vi "MainPageView.vi"() -> ()   [LabVIEW 2019]
uses:
  5219f83a-bb3a-43cd-b5ef-a6428703de02.vi
  bfe8fdff-ee4d-4ca5-9305-d53f92f2cf8d.vi
  e43f5a57-97c3-4510-b462-1dcb9a512c17.vi
  53e623ed-4a67-4f72-830e-33223b212eec.vi
  eefd14c2-1e60-472f-994b-7173b29c75b6.vi
  318ac530-f13b-4ebc-a1dc-b4da8ab9507f.vi
  911cadfa-6fc0-46bf-988e-f112db61373a.vi
  c961a98e-d49d-4477-bf1b-ce74dc2a816e.vi
  <vilib>/numeric/Random Number (Range) U64.vi
  <vilib>/numeric/sub_Random U32.vi
panel:
  in  "反馈延迟":u32=5 caption="侦听反馈延迟" max=5000 format="%.0f ms"
  in  "启用反馈？":bool
  in  "主发等待":u32=5 caption="发送后等待反馈" min=5 max=10000 format="%.0f ms"
  in  "等待延迟":u32=5 caption="侦听等待频率" min=5 max=5000 format="%.0f ms"
  out "循环引用":refnum<vi>
  out "计算后字符串":string
  out "预览":string
  in  "末尾":bool=TRUE
  in  "发送":bool
  in  "发送输入":string
  in  "寄存器重置":T1={"重置模式"=enum."址值一致", "数量"=1500, "值"=0}
  in  "清除记录":bool
  in  "清除显示":bool
  in  "寄存器重置":bool
  in  "选项卡":enum32{"被询问接收显示", "主动命令发收显示", "备注/解释/其它"}(tab)
  out "16":string[][](table) caption="功能码 16（0X10）"
  out "06":string[][](table) caption="功能码 06"
  out "03":string[][](table) caption="功能码 03"
  out "错误报文":string[][](table) caption="MB RTU 解析失败/其它 报文"
  in  "03去重":bool=TRUE caption="03指令去重？"
  out "主动接收":string[][](table) caption="接收"
  out "主动发送":string[][](table) caption="发送"
  out "连接通讯状态":bool
  out "报文流水显示":string
  in  "记录上限设置":u16=200 format="%d 条"
  out "模拟寄存器":u16[](array[numeric])
  out "连接提示":string
  out "连接模式":string
  out "显示连接":string
  in  "停止":bool
  # "发送时末尾添加?"
  # "+0"
  # "+5"
  # "+10"
  # "+15"
  # "ModbusRTU\n内置解析范围，当前针对功能码：03 06 16(十进制数)\n接收只针对询问报文的拆解，其它类型会被划分为未知命令\n\n示例格式(00代表U8字符，0000即U16字符，十六进制字符串显示)\n03询问：    01          03        0000         0001        XXXX \n            通讯地址  功能码  寄存器地址  需求数据量  CRC16\n03反馈：    01          03          00           0000 ... 0000         XXXX \n            通讯地址  功能码  数据字节量  数据段(根据询问反馈)  CRC16\n    **字节量代表U8数量，是数据量（U16字）的两倍。\n06下发/反馈  一致\n                01         06          0000      0000    XXXX\n            通讯地址  功能码  寄存器地址  写入值  CRC16\n16下发\n               01           10        0000        0001        02        0000     XXXX\n            通讯地址  功能码  寄存器地址  数据量  数据字节量  数据段  CRC16 \n16反馈\n               01          10        0000       0001    XXXX\n           通讯地址  功能码  寄存器地址  数据量  CRC16\n\n接收报文解析，只针对于询问/下发做拆解反馈"
  # "关于几个时间设置说明\n  通讯侦听部分是由\n    被动侦听-被动反馈-*主动发送命令-*主动命令反馈\n*指只有当前选中的连接执行，且无命令会忽略\n侦听等待频率-被动侦听等待超时设置\n发送后等待反馈-发送命令后等待反馈超时设置\n\n串口自发自收情况下，发送后无法获取反馈，需要测试修改\n正在测试中"
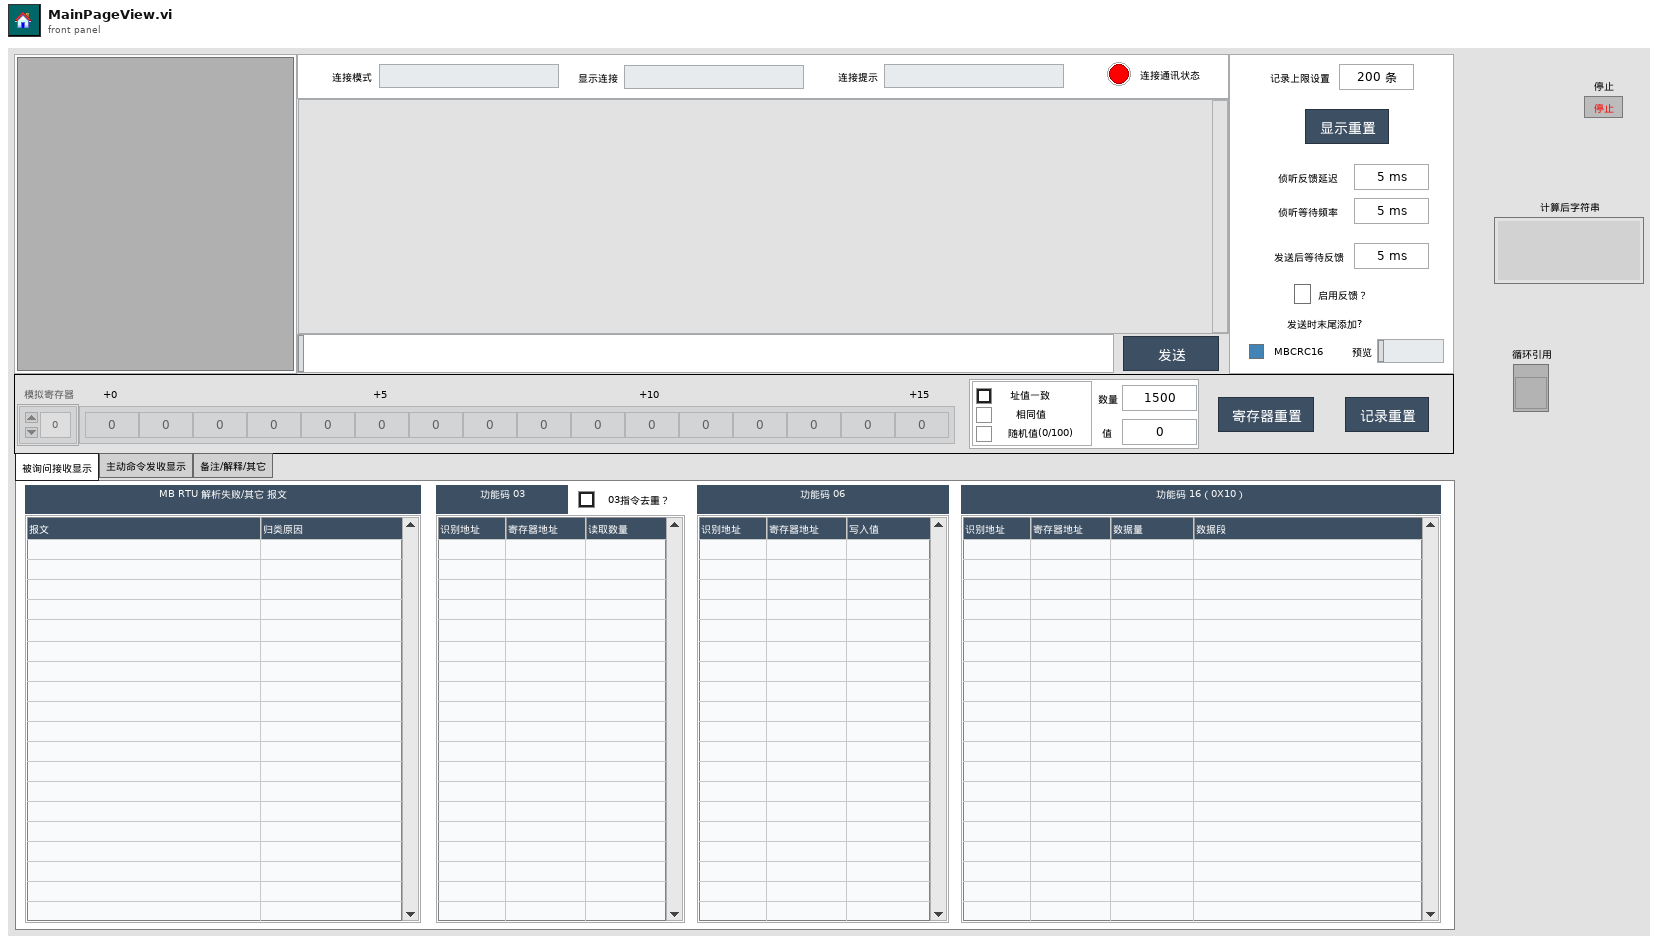
[diagram p1: front panel]
types:
  T1 = cluster{"重置模式":enum32{"址值一致", "相同值", "随机值(0/100)"}, "数量":u16, "值":u16}
  T2 = typedef "队列枚举.ctl" = enum16{"ini", "读", "写"}
  T3 = cluster{"识别名称":string, "记录":cluster{"通讯状态":bool, "记录上限":dbl, "报文记录":string[]}}
  T4 = enum16{"ini", "增", "删", "查", "改-通讯状态", "改-记录上限", "增-报文", "清空报文记录", "清空全部记录"}
  T5 = enum8{"Enabled", "Disabled", "Disabled and Grayed Out"}
  T6 = cluster{"无记录?":bool, "记录":cluster{"通讯状态":bool, "记录上限":dbl, "报文记录":string[][], "03类（被收）":string[], "06类（被收）":string[], "16类（被收）":string[], "主动发送记录":string[][], "主动接收记录":string[][], "无法识别记录":string[][]}}
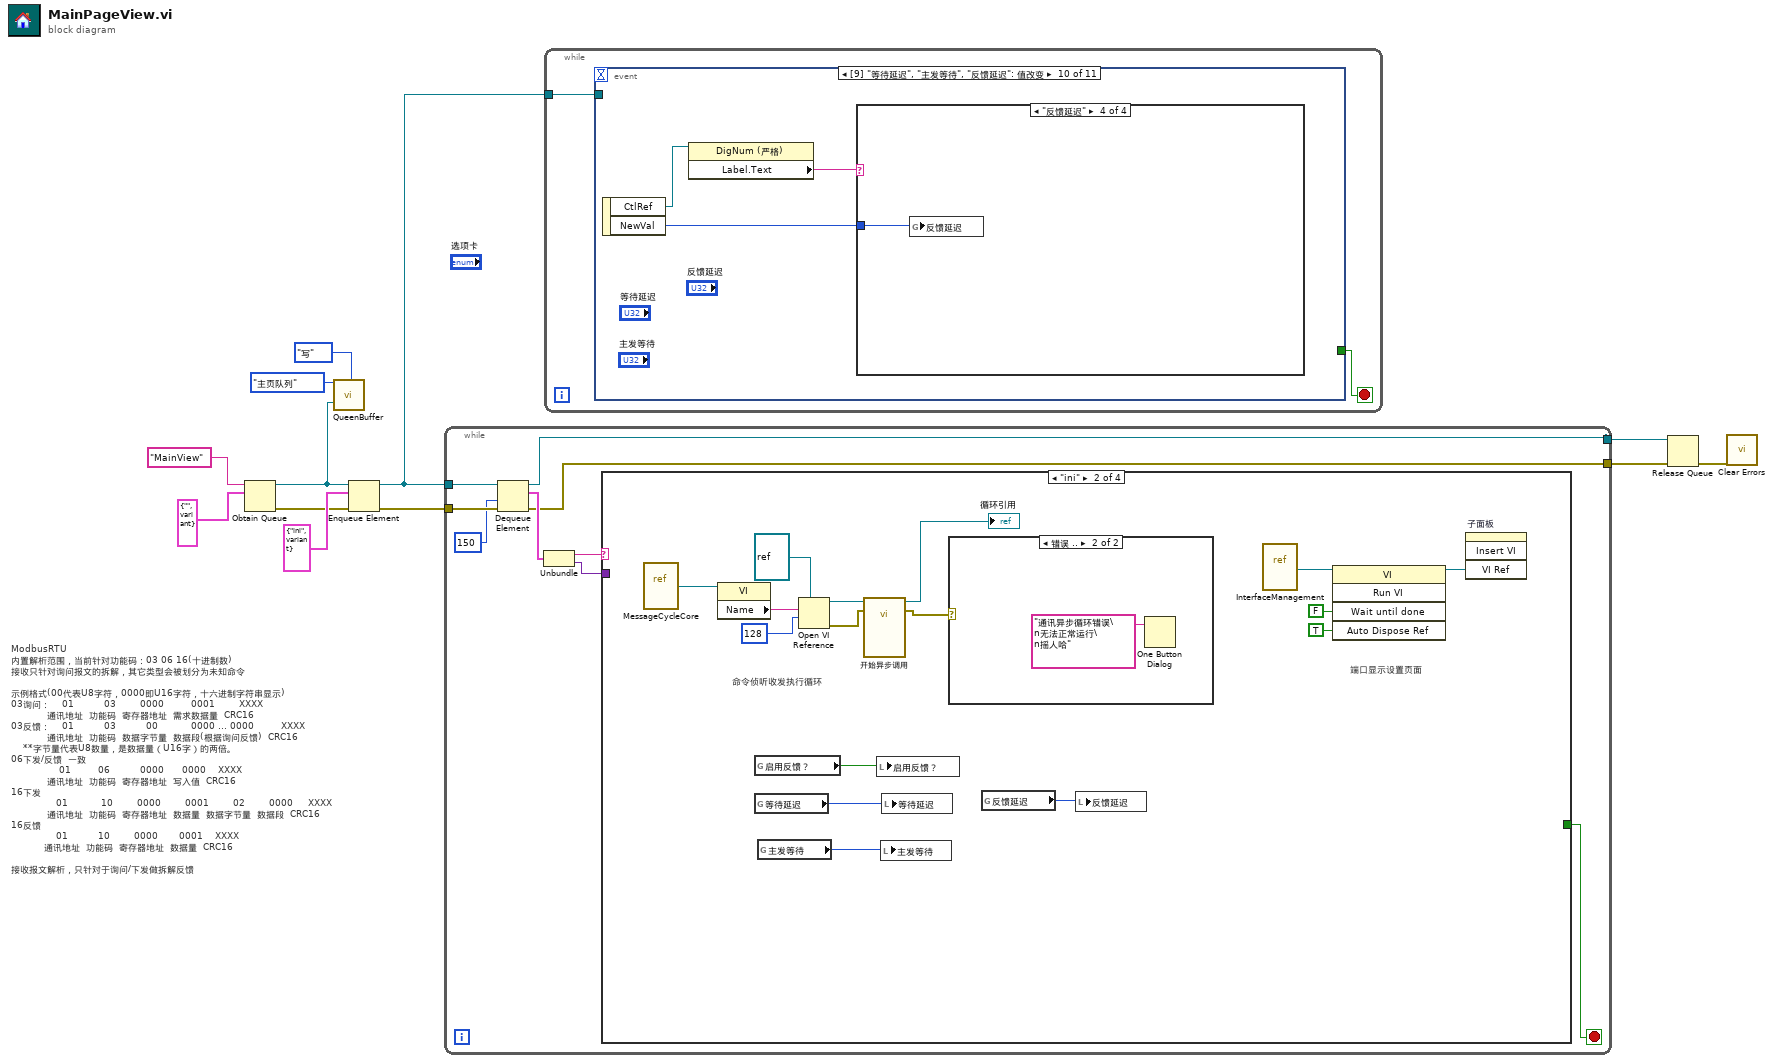
[diagram p0: block diagram]
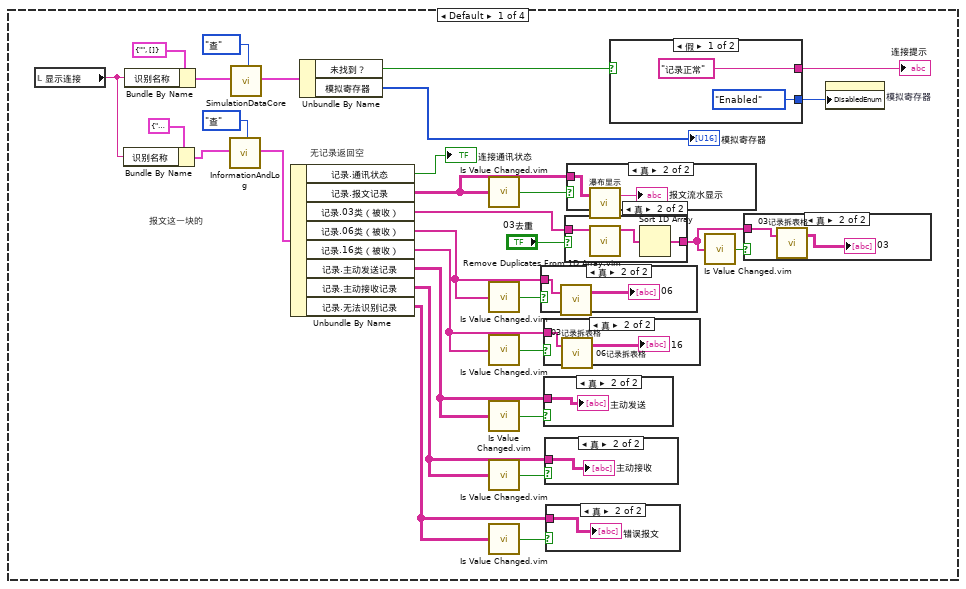
[diagram p2: hidden frame]
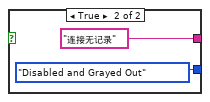
[diagram p11: hidden frame]
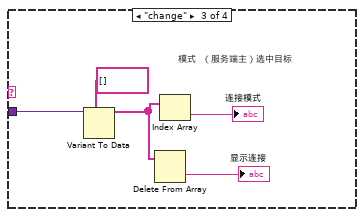
[diagram p13: hidden frame]
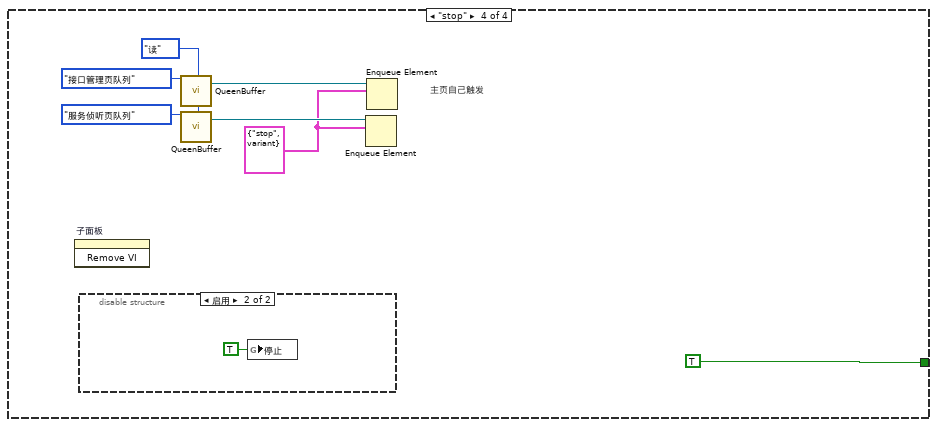
[diagram p14: hidden frame]
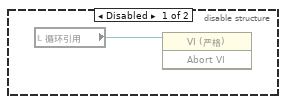
[diagram p15: hidden frame]
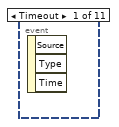
[diagram p16: hidden frame]
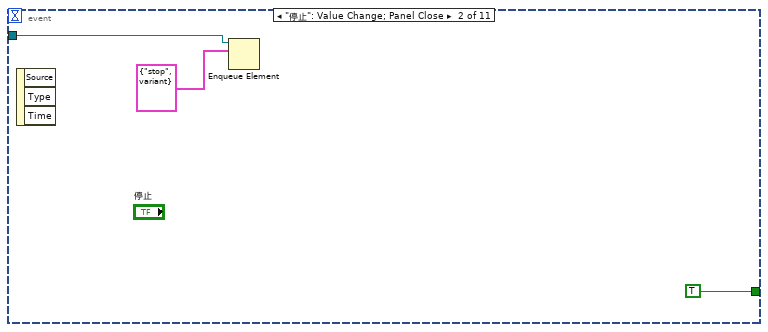
[diagram p17: hidden frame]
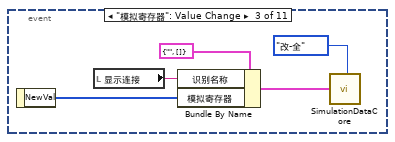
[diagram p18: hidden frame]
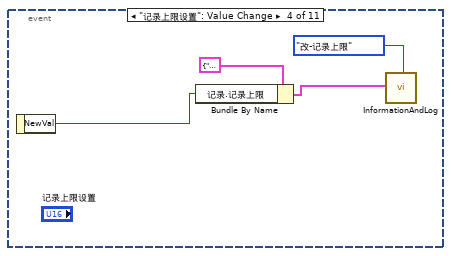
[diagram p19: hidden frame]
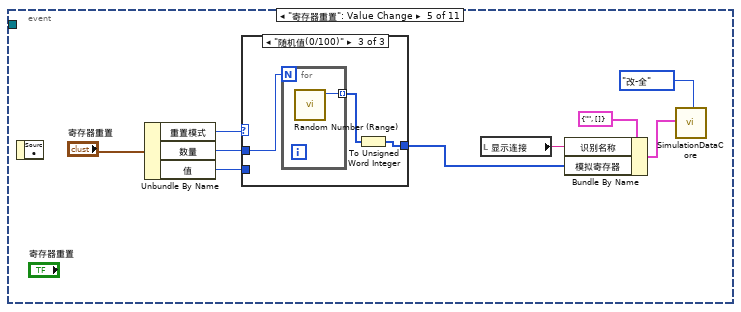
[diagram p20: hidden frame]
diagram:
  # "ModbusRTU\n内置解析范围，当前针对功能码：03 06 16(十进制数)\n接收只针对询问报文的拆解，其它类型会被划分为未知命令\n\n示例格式(00代表U8字符，0000即U16字符，十六进制字符串显示)\n03询问：    01          03        0000         0001        XXXX \n            通讯地址  功能码  寄存器地址  需求数据量  CRC16\n03反馈：    01          03          00           0000 ... 0000         XXXX \n            通讯地址  功能码  数据字节量  数据段(根据询问反馈)  CRC16\n    **字节量代表U8数量，是数据量（U16字）的两倍。\n06下发/反馈  一致\n                01         06          0000      0000    XXXX\n            通讯地址  功能码  寄存器地址  写入值  CRC16\n16下发\n               01           10        0000        0001        02        0000     XXXX\n            通讯地址  功能码  寄存器地址  数据量  数据字节量  数据段  CRC16 \n16反馈\n               01          10        0000       0001    XXXX\n           通讯地址  功能码  寄存器地址  数据量  CRC16\n\n接收报文解析，只针对于询问/下发做拆解反馈"
  n1 = Obtain Queue(name (unnamed)="MainView" ("名称（未命名）"), element data type=cluster{string, variant} {"", variant}) -> (queue out=w1:refnum<queue>, error out=w4:errorcluster)  [unwired: 3 in, 1 out]
  n2 = call "QueenBuffer.vi"("名称"=enum16{"接口管理页队列", "服务侦听页队列", "主页队列"}."主页队列", "目标队列输入"=w1, "操作"=队列枚举."写") -> ()  [unwired: 16 in, 1 out]
  n3 = Enqueue Element(queue=w1, element=cluster{string, variant} {"ini", variant} ("元素"), error in (no error)=w4) -> (queue out=w11:refnum<queue>, error out=w10:errorcluster)  [unwired: 1 in, 1 out]
  n4 = while {
    tunnel: w11 -> [w21]
    tunnel: w10 -> [w20]
    tunnel: [w16] -> w9
    tunnel: [w15] -> w8
    stop <- w14 stop-if-true
    n5 = Dequeue Element(queue=w21, timeout in ms (-1)=150 ("超时毫秒(-1)"), error in (no error)=w20) -> (queue out=w16:refnum<queue>, element=w19:cluster{string, variant}, error out=w15:errorcluster)  [unwired: 1 out]
    n6 = Unbundle(w19) -> (w18:string, w17:variant)
    n7 = case shown="\"ini\"" w18 {
      tunnel: w17 -> [_ _ w92 _]
      tunnel: [_ _ _ TRUE ("停止")] -> w14
      frame Default {
        # "无记录返回空"
        # "报文这一块的"
        n8 = local read "显示连接"() -> (w40:string)
        n9 = Bundle By Name(cluster=T3 {"识别名称"="", "记录"={"通讯状态"=FALSE, "记录上限"=0.0, "报文记录"=[]}} ("配置信息"), "识别名称"=w40) -> (w41:T3)
        n10 = Bundle By Name(cluster=cluster{"识别名称":string, "模拟寄存器":u16[]} {"识别名称"="", "模拟寄存器"=[]} ("配置信息"), "识别名称"=w40) -> (w49:cluster{"识别名称":string, "模拟寄存器":u16[]})
        n11 = call "InformationAndLog.vi"("配置信息"=w41, "模拟数据枚举"=T4."查") -> ("结果反馈"=w39:T6)  [unwired: 16 in, 1 out]
        n12 = call "SimulationDataCore.vi"("配置信息"=w49, "模拟数据枚举"=enum16{"ini", "增", "删", "查", "改-全", "改-部分"}."查") -> ("结果"=w48:cluster{"未找到？":bool, "模拟寄存器":u16[]})  [unwired: 16 in, 1 out]
        n13 = Unbundle By Name(w39) -> ("记录.通讯状态"=→"连接通讯状态":bool, "记录.报文记录"=w36:string[][], "记录.03类（被收）"=w33:string[], "记录.06类（被收）"=w30:string[], "记录.16类（被收）"=w28:string[], "记录.主动发送记录"=w24:string[][], "记录.主动接收记录"=w22:string[][], "记录.无法识别记录"=w23:string[][])
        n14 = Unbundle By Name(w48) -> ("未找到？"=w47:bool, "模拟寄存器"=→"模拟寄存器":u16[])
        n15 = call "Is Value Changed.vim"("value"=w36) -> ("changed or first call?"=w37:bool)
        n16 = call "Is Value Changed.vim"("value"=w30) -> ("changed or first call?"=w31:bool)
        n17 = call "Is Value Changed.vim"("value"=w28) -> ("changed or first call?"=w29:bool)
        n18 = call "Is Value Changed.vim"("value"=w24) -> ("changed or first call?"=w27:bool)
        n19 = call "Is Value Changed.vim"("value"=w22) -> ("changed or first call?"=w26:bool)
        n20 = call "Is Value Changed.vim"("value"=w23) -> ("changed or first call?"=w25:bool)
        n21 = case shown="真" w31 {
          tunnel: w30 -> [_ w57]
          frame False {
          }
          frame True {
            n22 = call "03记录拆表格.vi"("03类（被收）"=w57) -> ("拆分显示（主页）"=→"06":string[][])  [unwired: 18 in]
          }
        }
        n23 = case shown="真" w29 {
          tunnel: w28 -> [_ w56]
          frame False {
          }
          frame True {
            n24 = call "06记录拆表格.vi"("16类（被收）"=w56) -> ("拆分显示（主页）"=→"16":string[][])  [unwired: 18 in]
          }
        }
        n25 = case shown="真" w27 {
          tunnel: w24 -> [_ w54]
          frame False {
          }
          frame True {
            "主动发送" <- w54
          }
        }
        n26 = case shown="真" w26 {
          tunnel: w22 -> [_ w53]
          frame False {
          }
          frame True {
            "主动接收" <- w53
          }
        }
        n27 = case shown="真" w25 {
          tunnel: w23 -> [_ w52]
          frame False {
          }
          frame True {
            "错误报文" <- w52
          }
        }
        n28 = case shown="真" "03去重" {
          tunnel: w33 -> [w59 w61]
          tunnel: [w59 w60] -> w32
          frame False {
          }
          frame True {
            n29 = call "Remove Duplicates From 1D Array.vim"("array"=w61) -> ("array with duplicates removed"=w62:string[])  [unwired: 10 in]
            n30 = Sort 1D Array(array=w62) -> (sorted array=w60:string[])
          }
        }
        n31 = case shown="真" w37 {
          tunnel: w36 -> [_ w66]
          frame False {
          }
          frame True {
            n32 = call "瀑布显示.vi"("报文信息记录"=w66) -> ("显示"=→"报文流水显示":string)  [unwired: 18 in]
          }
        }
        n33 = case shown="假" w47 {
          tunnel: ["记录正常" "连接无记录"] -> w46
          tunnel: [T5."Enabled" ("禁用") T5."Disabled and Grayed Out" ("禁用")] -> w44
          frame False {
          }
          frame True {
          }
        }
        "连接提示" <- w46
        n34 = call "Is Value Changed.vim"("value"=w32) -> ("changed or first call?"=w35:bool)
        n35 = case shown="真" w35 {
          tunnel: w32 -> [_ w64]
          frame False {
          }
          frame True {
            n36 = call "03记录拆表格.vi"("03类（被收）"=w64) -> ("拆分显示（主页）"=→"03":string[][])  [unwired: 18 in]
          }
        }
        n37 = property on="模拟寄存器" class="Arr (严格)"("DisabledEnum"=w44) -> ()  [unwired: 2 in, 2 out]
      }
      frame "ini" {
        # "命令侦听收发执行循环"
        # "端口显示设置页面"
        n38 = vi-ref "MessageCycleCore.vi"() -> (w83:refnum<vi>)
        n39 = property class="VI"(reference=w83) -> ("Name"=w86:string)  [unwired: 1 in, 2 out]
        n40 = global read "全局-被反馈配置.vi" "启用反馈？"() -> (w72:bool)
        n41 = global read "全局-配置识别.vi" "等待延迟"() -> (w74:u32)
        n42 = global read "全局-配置识别.vi" "主发等待"() -> (w73:u32)
        n43 = Open VI Reference(type specifier VI Refnum (for type only)=refnum<vi> refnum ("类型说明符VI引用句柄（仅用于类型）"), vi path=w86, options=128 ("选项")) -> (vi reference=w82:refnum<vi>, error out=w81:errorcluster)  [unwired: 3 in]
        n44 = call-by-ref "开始异步调用"(reference=w82, error in=w81) -> (reference out=→"循环引用":refnum<vi>, error out=w80:errorcluster)  [unwired: 20 in]
        n45 = local write "启用反馈？"(w72) -> ()
        n46 = local write "主发等待"(w73) -> ()
        n47 = local write "等待延迟"(w74) -> ()
        n48 = case shown="错误 .." w80 {
          frame No Error {
          }
          frame Error {
            n49 = One Button Dialog(message="通讯异步循环错误\n无法正常运行\n摇人哈" ("消息")) -> ()  [unwired: 1 in, 1 out]
          }
        }
        n50 = global read "全局-配置识别.vi" "反馈延迟"() -> (w71:u32)
        n51 = local write "反馈延迟"(w71) -> ()
        n52 = vi-ref "InterfaceManagement.vi"() -> (w78:refnum<vi>)
        n53 = invoke class="VI" method="Run VI"(reference=w78, "Wait until done"=FALSE ("结束前等待"), "Auto Dispose Ref"=TRUE ("自动销毁引用")) -> (reference out=w75:refnum<vi>)  [unwired: 2 in, 4 out]
        n54 = invoke on="子面板" class="SubPnl" method="Insert VI"("VI Ref"=w75) -> ()  [unwired: 3 in, 4 out]
      }
      frame "change" {
        # "模式  （服务端主）选中目标"
        n55 = Variant To Data(type=string[] [], Variant=w92) -> (data=w90:string[])  [unwired: 1 in, 1 out]
        n56 = Delete From Array(array=w90) -> (deleted portion=→"显示连接":string)  [unwired: 2 in, 1 out]
        n57 = Index Array(array=w90) -> (element=→"连接模式":string)  [unwired: 1 in]
      }
      frame "stop" {
        w95 = 队列枚举."读" ("操作")
        w96 = cluster{string, variant} {"stop", variant} ("元素")
        # "主页自己触发"
        n58 = invoke on="子面板" class="SubPnl" method="Remove VI"() -> ()  [unwired: 3 in, 3 out]
        n59 = disable-structure shown="启用" {
          frame Disabled {
            n60 = local read "循环引用"() -> (w100:refnum<vi>)
            n61 = invoke class="VI (严格)" method="Abort VI"(reference=w100) -> ()  [unwired: 2 in, 3 out]
          }
          frame Enabled {
            n62 = global write "全局-配置识别.vi" "停止"(TRUE ("停止")) -> ()
          }
        }
        n63 = call "QueenBuffer.vi"("名称"=enum16{"接口管理页队列", "服务侦听页队列", "主页队列"}."接口管理页队列", "操作"=w95) -> ("目标队列"=w98:refnum<queue>)  [unwired: 17 in]
        n64 = call "QueenBuffer.vi"("名称"=enum16{"接口管理页队列", "服务侦听页队列", "主页队列"}."服务侦听页队列", "操作"=w95) -> ("目标队列"=w97:refnum<queue>)  [unwired: 17 in]
        n65 = Enqueue Element(queue=w97, element=w96) -> ()  [unwired: 2 in, 3 out]
        n66 = Enqueue Element(queue=w98, element=w96) -> ()  [unwired: 2 in, 3 out]
      }
    }
  }
  n67 = while {
    tunnel: w11 -> [w102]
    stop <- w103 stop-if-true
    n68 = event shown="[9] \"等待延迟\", \"主发等待\", \"反馈延迟\": 值改变" {
      selector: _ -> [_ _ _ _ _ _ _ _ _ _ _]
      dyn-events: _ -> [_ _ _ _ _ _ _ _ _ _ _]
      timeout: _ -> [_ _ _ _ _ _ _ _ _ _ _]
      tunnel: [_ TRUE ("停止") _ _ _ _ _ _ _ _ _] -> w103
      tunnel: w102 -> [_ w105 _ _ _ _ _ _ _ _ _]
      event Timeout {
        n69 = event-data() -> ()  [unwired: 1 in, 3 out]
      }
      event "停止": Value Change; Panel Close {
        n70 = event-data() -> ()  [unwired: 1 in, 3 out]
        n71 = Enqueue Element(queue=w105, element=cluster{string, variant} {"stop", variant} ("元素")) -> ()  [unwired: 2 in, 3 out]
      }
      event "模拟寄存器": Value Change {
        n72 = event-data() -> ("NewVal"=w108:u16[])  [unwired: 1 in]
        n73 = local read "显示连接"() -> (w110:string)
        n74 = Bundle By Name(cluster=cluster{"识别名称":string, "模拟寄存器":u16[]} {"识别名称"="", "模拟寄存器"=[]} ("配置信息"), "识别名称"=w110, "模拟寄存器"=w108) -> (w107:cluster{"识别名称":string, "模拟寄存器":u16[]})
        n75 = call "SimulationDataCore.vi"("配置信息"=w107, "模拟数据枚举"=enum16{"ini", "增", "删", "查", "改-全", "改-部分"}."改-全") -> ()  [unwired: 16 in, 2 out]
      }
      event "记录上限设置": Value Change {
        n76 = event-data() -> ("NewVal"=w114:u16)  [unwired: 1 in]
        n77 = Bundle By Name(cluster=T3 {"识别名称"="", "记录"={"通讯状态"=FALSE, "记录上限"=0.0, "报文记录"=[]}} ("配置信息"), "记录.记录上限"=w114) -> (w113:T3)
        n78 = call "InformationAndLog.vi"("配置信息"=w113, "模拟数据枚举"=T4."改-记录上限") -> ()  [unwired: 16 in, 2 out]
      }
      event "寄存器重置": Value Change {
        n79 = event-data() -> ()  [unwired: 1 in, 1 out]
        n80 = Unbundle By Name("寄存器重置") -> ("重置模式"=w123:enum32{"址值一致", "相同值", "随机值(0/100)"}, "数量"=w117:u16, "值"=w116:u16)
        n81 = case shown="\"随机值(0/100)\"" w123 {
          tunnel: [w125 w129 w133] -> w118
          tunnel: w117 -> [w126 w131 w134]
          tunnel: w116 -> [_ w130 _]
          frame "址值一致", Default {
            n82 = for {
              N: w126 -> [_]
              tunnel: [w127] -> w125 mode=indexing
              i -> [w128]
              n83 = To Unsigned Word Integer(number=w128) -> (unsigned 16bit integer=w127:u16)
            }
          }
          frame "相同值" {
            n84 = Initialize Array(w130, w131) -> (w129:u16[])
          }
          frame "随机值(0/100)" {
            n85 = for {
              N: w134 -> [_]
              tunnel: [w135] -> w132 mode=indexing
              n86 = call-poly <vilib>:"Random Number (Range).vi"() -> ("number"=w135:u64)  [unwired: 11 in]
            }
            n87 = To Unsigned Word Integer(number=w132) -> (unsigned 16bit integer=w133:u16[])
          }
        }
        n88 = local read "显示连接"() -> (w121:string)
        n89 = Bundle By Name(cluster=cluster{"识别名称":string, "模拟寄存器":u16[]} {"识别名称"="", "模拟寄存器"=[]} ("配置信息"), "识别名称"=w121, "模拟寄存器"=w118) -> (w119:cluster{"识别名称":string, "模拟寄存器":u16[]})
        n90 = call "SimulationDataCore.vi"("配置信息"=w119, "模拟数据枚举"=enum16{"ini", "增", "删", "查", "改-全", "改-部分"}."改-全") -> ()  [unwired: 16 in, 2 out]
      }
      event "清除显示": Value Change {
        n91 = event-data() -> ()  [unwired: 1 in, 1 out]
        n92 = local read "显示连接"() -> (w138:string)
        n93 = Bundle By Name(cluster=T3 {"识别名称"="", "记录"={"通讯状态"=FALSE, "记录上限"=0.0, "报文记录"=[]}} ("配置信息"), "识别名称"=w138) -> (w137:T3)
        n94 = call "InformationAndLog.vi"("配置信息"=w137, "模拟数据枚举"=T4."清空报文记录") -> ()  [unwired: 16 in, 2 out]
      }
      event "清除记录": Value Change {
        n95 = event-data() -> ()  [unwired: 1 in, 6 out]
        n96 = local read "显示连接"() -> (w143:string)
        n97 = Bundle By Name(cluster=T3 {"识别名称"="", "记录"={"通讯状态"=FALSE, "记录上限"=0.0, "报文记录"=[]}} ("配置信息"), "识别名称"=w143) -> (w142:T3)
        n98 = call "InformationAndLog.vi"("配置信息"=w142, "模拟数据枚举"=T4."清空全部记录") -> ()  [unwired: 16 in, 2 out]
      }
      event "发送": Value Change {
        n99 = event-data() -> ()  [unwired: 1 in, 1 out]
        n100 = local read "末尾"() -> (w146:bool)
        n101 = case shown="真" w146 {
          tunnel: "发送输入" -> [w148 w151]
          tunnel: [w148 w149] -> w144
          frame False {
          }
          frame True {
            n102 = local read "预览"() -> (w150:string)
            n103 = Concatenate Strings(w151, w150) -> (w149:string)
          }
        }
        n104 = call "发送报文存储-功能全局.vi"("报文输入"=w144, "枚举"=enum16{"ini", "读", "写"}."写") -> ()  [unwired: 17 in, 1 out]
      }
      event "发送输入": Value Change {
        n105 = event-data() -> ("NewVal"=w154:string)  [unwired: 1 in]
        n106 = case shown="真" "末尾" {
          tunnel: w154 -> [_ w162]
          tunnel: [_ w156] -> w153
          frame False {
          }
          frame True {
            n107 = String To Byte Array(string=w162) -> (unsigned byte array=w161:u8[])
            n108 = call "CRC计算.vi"("无校验U8数组"=w161) -> ("计算后字符串"=→"计算后字符串":string, "CRC值"=w160:u16)  [unwired: 17 in]
            n109 = Split Number(x=w160) -> (hi(x)=w158:u8, lo(x)=w159:u8)
            n110 = Build Array(w159, w158) -> (w157:u8[])
            n111 = Byte Array To String(unsigned byte array=w157) -> (string=w156:string)
          }
        }
        "预览" <- w153
      }
      event "等待延迟", "主发等待", "反馈延迟": Value Change {
        n112 = event-data() -> ("CtlRef"=w165:refnum<vi>, "NewVal"=w163:u32)  [unwired: 1 in]
        n113 = property class="DigNum (严格)"(reference=w165) -> ("Label.Text"=w164:string)  [unwired: 1 in, 2 out]
        n114 = case shown="\"反馈延迟\"" w164 {
          tunnel: w163 -> [_ w166 w167 w168]
          frame Default {
          }
          frame "等待延迟" {
            n115 = global write "全局-配置识别.vi" "等待延迟"(w166) -> ()
          }
          frame "主发等待" {
            n116 = global write "全局-配置识别.vi" "主发等待"(w167) -> ()
          }
          frame "反馈延迟" {
            n117 = global write "全局-配置识别.vi" "反馈延迟"(w168) -> ()
          }
        }
      }
      event "启用反馈？": Value Change {
        n118 = event-data() -> ("NewVal"=w169:bool)  [unwired: 1 in]
        n119 = global write "全局-被反馈配置.vi" "启用反馈？"(w169) -> ()
      }
    }
  }
  n120 = Release Queue(queue=w9, error in (no error)=w8) -> (error out=w7:errorcluster)  [unwired: 1 in, 2 out]
  n121 = call <vilib>:"Clear Errors.vi"("error in (no error)"=w7) -> ()  [unwired: 5 in, 2 out]
